vi "Get Sender.vi"(8 "error in (no error)":errorcluster caption="错误输入（无错误）", 11 "Message输入":refnum<class "Message.lvclass">) -> (0 "error out":errorcluster caption="错误输出", 2 "Sender":string, 3 "Message输出":refnum<class "Message.lvclass">)   [LabVIEW 2011, in "Message.lvclass"]
uses:
  Message.lvclass
  Message.lvclass/Message.ctl
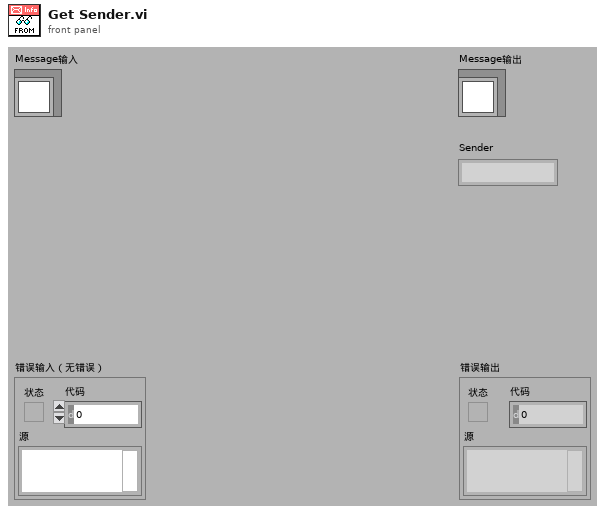
[diagram p1: front panel]
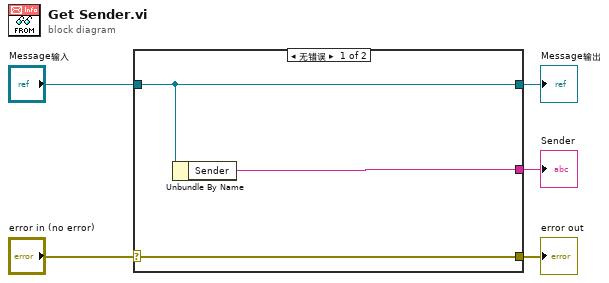
[diagram p0: block diagram]
diagram:
  n1 = case shown="无错误" "error in (no error)" {
    selector: "error in (no error)" -> [w8 w9]
    tunnel: [w8 w9] -> w4
    tunnel: [w7 w10] -> w2
    tunnel: "Message输入" -> [w7 w10]
    tunnel: [w6 _] -> w1
    frame No Error {
      n2 = Unbundle By Name(w7) -> ("Sender"=w6:string)
    }
    frame Error {
    }
  }
  "error out" <- w4
  "Message输出" <- w2
  "Sender" <- w1
